vi "DBTester6.vi"() -> ()   [LabVIEW 2015]
uses:
  BERTTA.dll
panel:
  in  "new element/subarray":string[](array[string])
  in  "col 2":i32=3
  out "Table":string[][](table)
  in  "col":i32=2
  out "Mettler":dynamicdata(graph)
  in  "Device port":i32=6
  out "Weight":dbl
  out "Weight 2":dbl
  in  "Device port 2":i32=2
  out "rc":i32
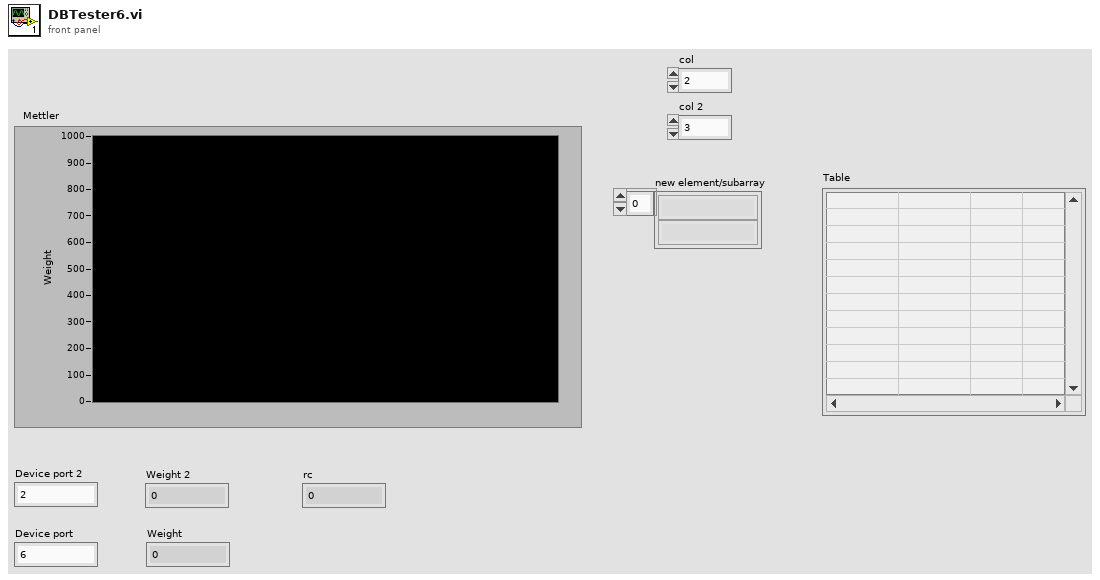
[diagram p1: front panel]
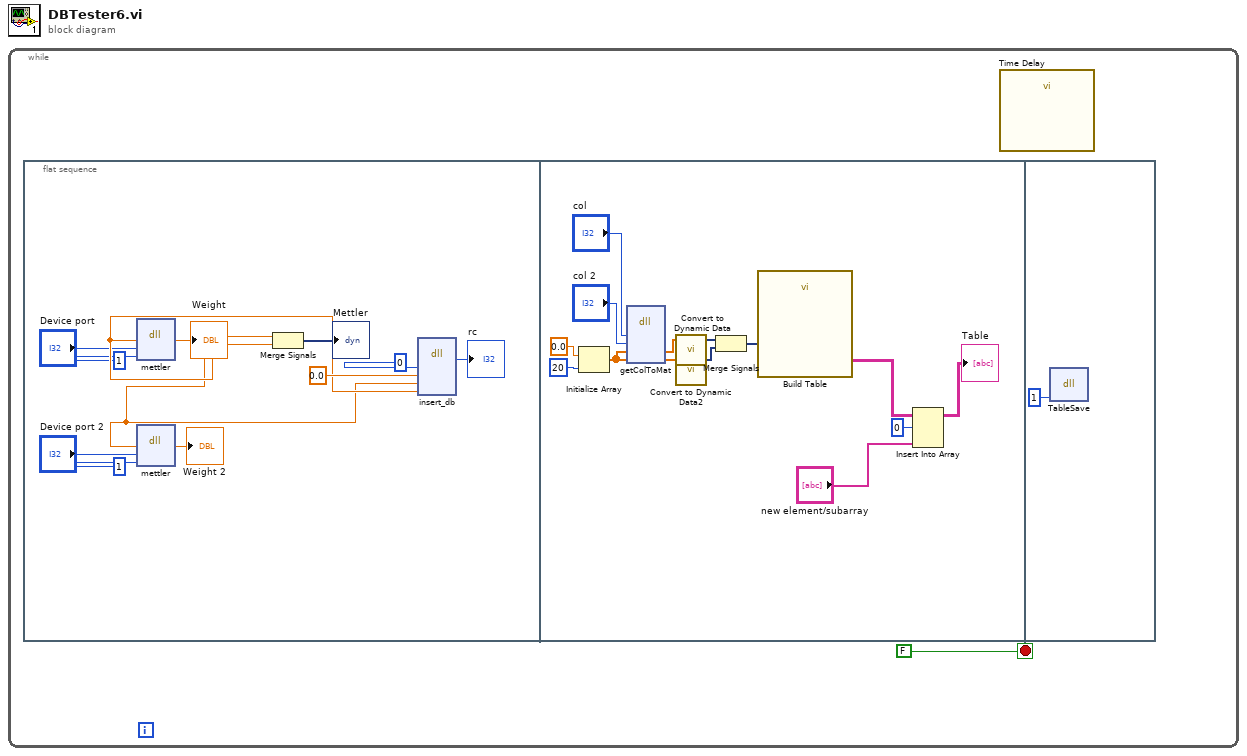
[diagram p0: block diagram]
diagram:
  n1 = while {
    stop <- FALSE stop-if-true
    n2 = flat-sequence {
      frame #0 {
        n3 = dll-call lib="C:/Users/xlaraser/Documents/Visual Studio 2017/Projects/Bertta/BERTTA/Debug/BERTTA.dll" fn="mettler"("port"="Device port", "msg"=1) -> ("return type"=w9:dbl)  [unwired: 5 in, 2 out]
        "Weight" <- w9
        n4 = dll-call lib="C:/Users/xlaraser/Documents/Visual Studio 2017/Projects/Bertta/BERTTA/Debug/BERTTA.dll" fn="mettler"("port"="Device port 2", "msg"=1) -> ("return type"=w8:dbl)  [unwired: 5 in, 2 out]
        "Weight 2" <- w8
        n5 = Merge Signals(w8, w9) -> (→"Mettler":dynamicdata)
        n6 = dll-call lib="C:/Users/xlaraser/Documents/Visual Studio 2017/Projects/Bertta/BERTTA/Debug/BERTTA.dll" fn="insert_db"("heidolph"=0, "lauda"=0.0, "mettler1"=w8, "mettler2"=w9) -> ("return type"=→"rc":i32)  [unwired: 7 in, 2 out]
      }
      frame #1 {
        n7 = Initialize Array(0.0 ("element"), 20 ("dimension size")) -> (w21:dbl[])
        n8 = dll-call lib="C:/Users/xlaraser/Documents/Visual Studio 2017/Projects/Bertta/BERTTA/Debug/BERTTA.dll" fn="getColToMat"("col1"="col", "col2"="col 2", "values1"=w21, "values2"=w21) -> ("values1"=w22:dbl[], "values2"=w18:dbl[])  [unwired: 6 in, 2 out]
        n9 = call "Convert to Dynamic Data"("Array"=w22) -> ("Dynamic Data Type"=w19:dynamicdata)  [unwired: 3 in]
        n10 = call "Convert to Dynamic Data2"("Array"=w18) -> ("Dynamic Data Type"=w17:dynamicdata)  [unwired: 3 in]
        n11 = Merge Signals(w19, w17) -> (w16:dynamicdata)
        n12 = call "Build Table"("Signals"=w16) -> ("Table"=w15:string[][])  [unwired: 4 in, 6 out]
        n13 = Insert Into Array(array=w15, index (row)=0, new element="new element/subarray") -> (→"Table":string[][])  [unwired: 1 in]
      }
      frame #2 {
        n14 = dll-call lib="C:/Users/xlaraser/Documents/Visual Studio 2017/Projects/Bertta/BERTTA/Debug/BERTTA.dll" fn="TableSave"("exec"=1) -> ()  [unwired: 5 in, 2 out]
      }
    }
    n15 = call "Time Delay"() -> ()  [unwired: 11 in, 1 out]
  }
